vi "Initialize.vi"(5 "Operation Interface in":refnum<class "Program Interface.lvclass">) -> (19 "Operation Interface out":refnum<class "Program Interface.lvclass">)   [LabVIEW 2016, in "Program Interface.lvclass"]
uses:
  Program Interface.lvclass
  Program Interface.lvclass/Program Interface.ctl
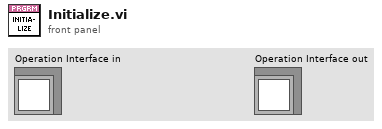
[diagram p1: front panel]
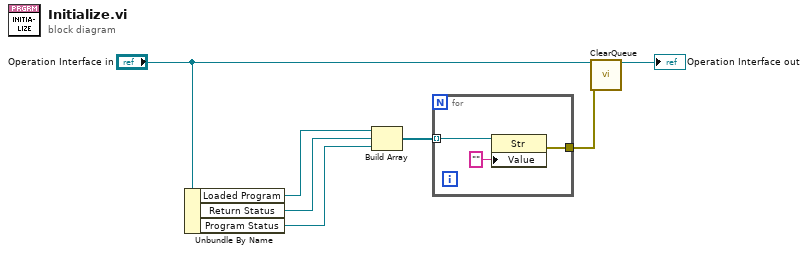
[diagram p0: block diagram]
diagram:
  n1 = Unbundle By Name("Operation Interface in") -> ("Loaded Program"=w7:refnum<vi>, "Return Status"=w6:refnum<vi>, "Program Status"=w5:refnum<vi>)
  n2 = Build Array(w7, w6, w5) -> (w4:refnum<vi>[])
  n3 = for {
    tunnel: w4 -> [w10] mode=indexing
    tunnel: [w8] -> w1
    n4 = property class="Str"(reference=w10, "Value"="") -> (error out=w8:errorcluster)  [unwired: 1 in, 1 out]
  }
  n5 = call "ClearQueue.vi"("Program Interface in"="Operation Interface in", "error in (no error)"=w1) -> ("Program Interface out"=→"Operation Interface out":refnum<class "Program Interface.lvclass">)  [unwired: 16 in, 1 out]
